vi "Autonomous Independent.vi"() -> ()   [LabVIEW 2012]
doc: "This VI is called when autonomous begins, and will automatically be terminated when autonomous ends. You can carry out timed or sensor driven robot movement independently without needing to return to the caller."
uses:
  Auto States.ctl
  <vilib>/Rock Robotics/WPI/Relay/WPI_RelayValue.ctl
  <vilib>/Rock Robotics/WPI/Solenoid/WPI_SolenoidValue.ctl
  Robot Global Data.vi
  <vilib>/Rock Robotics/WPI/RobotDrive/WPI_RobotDriveGetSetRefNum.vi
  <vilib>/Rock Robotics/WPI/Solenoid/WPI_SolenoidSetEnum.vi
  <vilib>/Rock Robotics/WPI/RobotDrive/WPI_RobotDriveArcadeDrive_Standard(NoSaturation).vi
panel:
  in  "Debug":bool
  in  "?":T1
  out "Current Movement, for debugging":T2 {"Y Joystick Value" scale=1.0..-1.0; "X Joystick Value" scale=-1.0..1.0}
  in  "Array of robot movements":T3(array[cluster]) {"Y Joystick Value" scale=1.0..-1.0; "X Joystick Value" scale=-1.0..1.0}
  # "Be sure to right-click and choose Data Operations>>Make Current Value default if you want to save the array values with the VI"
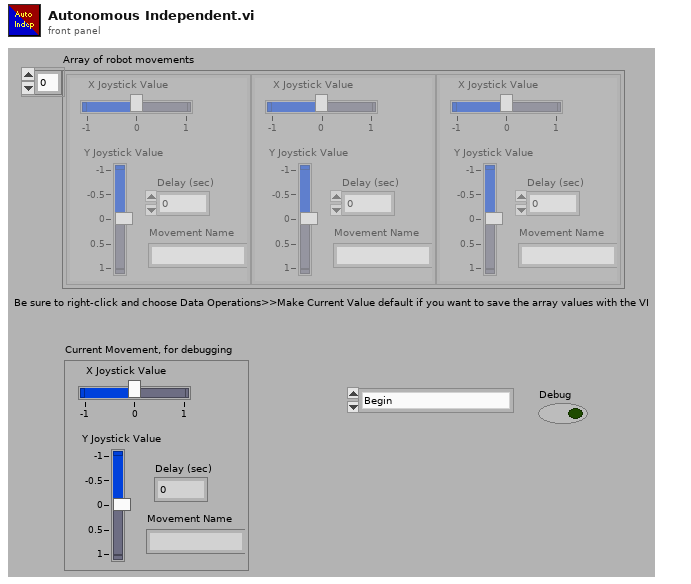
[diagram p1: front panel]
types:
  T1 = typedef "Auto States.ctl" = enum16{"Begin", "2 Top/Mid Goal", "3 Top/Mid Goal", "Drive to shoot", "Auto-Lock", "Spin 180 and Auto-Lock", "Drive Backwards", "Drive forward (Dump)", "Slow Shoot", "End"}
  T2 = cluster{"X Joystick Value":dbl, "Y Joystick Value":dbl, "Delay (sec)":dbl, "Movement Name":string}
  T3 = cluster{"X Joystick Value":dbl, "Y Joystick Value":dbl, "Delay (sec)":dbl, "Movement Name":string}[]
  T4 = typedef "WPI_RobotDriveDevRef.ctl" = cluster{"DevStatus":errorcluster, "Motors[]":T5[], "Square Inputs":bool, "Max Output":dbl, "Isochronous":bool}
  T5 = typedef "WPI_MotorControlDeviceRef.ctl" = cluster{"DeviceStatus":errorcluster, "Type":enum16{"PWM", "CAN"}, "PWM":cluster{"Digital Module":T6, "PWM Channel":T7, "DeadBand":T8}, "CAN":cluster{"Device Number":u8, "Control Mode":T9, "Semaphore":T10, "Max Vout":dbl}, "Invert":bool, "TransformRef":T11, "InvTransformRef":T11}
  T6 = typedef "FPGA_TypedefDigitalModule.ctl" = enum16{"Digital Module 1", "Digital Module 2"}
  T7 = typedef "FPGA_DIOPWMChannel.ctl" = enum8{"PWM 1", "PWM 2", "PWM 3", "PWM 4", "PWM 5", "PWM 6", "PWM 7", "PWM 8", "PWM 9", "PWM 10", "Invalid"}
  T8 = typedef "WPI_PWMDeadband.ctl" = cluster{"Name":string, "maxPositivePwm":i32, "minPositivePwm":i32, "centerPwm":i32, "maxNegativePwm":i32, "minNegativePwm":i32, "angularRange":u16}
  T9 = typedef "WPI_CANJaguar_ControlMode.ctl" = enum8{"Percent VBus", "Current", "Speed", "Position", "Voltage"}
  T10 = typedef "Semaphore RefNum" = refnum<k1>
  T11 = typedef "WPI_PWMTransform_ConPane.ctl" = refnum<vi>
  T12 = typedef "Auto State Selector.ctl" = enum16{"None", "Fire 2x", "Fire 3x", "Fire 3x from back", "Dump in low goal"}
  T13 = typedef "WPI_RelayValue.ctl" = enum16{"Off", "On", "Forward", "Reverse"}
  T14 = typedef "WPI_SolenoidValue.ctl" = enum16{"Off", "On", "Forward", "Reverse"}
  T15 = typedef "WPI_RelayDevRef.ctl" = cluster{"DevStatus":errorcluster, "Relay Channel":T16, "Digital Module":T6, "Relay Direction":T17}
  T16 = typedef "FPGA_DIORelayChannel.ctl" = enum8{"Relay 1", "Relay 2", "Relay 3", "Relay 4", "Relay 5", "Relay 6", "Relay 7", "Relay 8", "Invalid"}
  T17 = typedef "WPI_RelayDirection.ctl" = enum16{"Both directions", "Forward only", "Reverse only"}
  T18 = typedef "WPI_SolenoidDevRef.ctl" = cluster{"DevStatus":errorcluster, "Solenoid Module":T19, "Forward Solenoid Channel":T20, "Reverse Solenoid Channel":T20}
  T19 = typedef "FPGA_TypedefSolenoidModule.ctl" = enum16{"Solenoid Module 1", "Solenoid Module 2"}
  T20 = typedef "WPI_SolenoidChannel.ctl" = enum8{"Solenoid 1", "Solenoid 2", "Solenoid 3", "Solenoid 4", "Solenoid 5", "Solenoid 6", "Solenoid 7", "Solenoid 8", "Invalid"}
  T21 = cluster{"Center Position":cluster{"X":dbl, "Y":dbl}, "Distance (ft)":dbl, "Center":bool, "Top":bool, "Mid":bool}[]
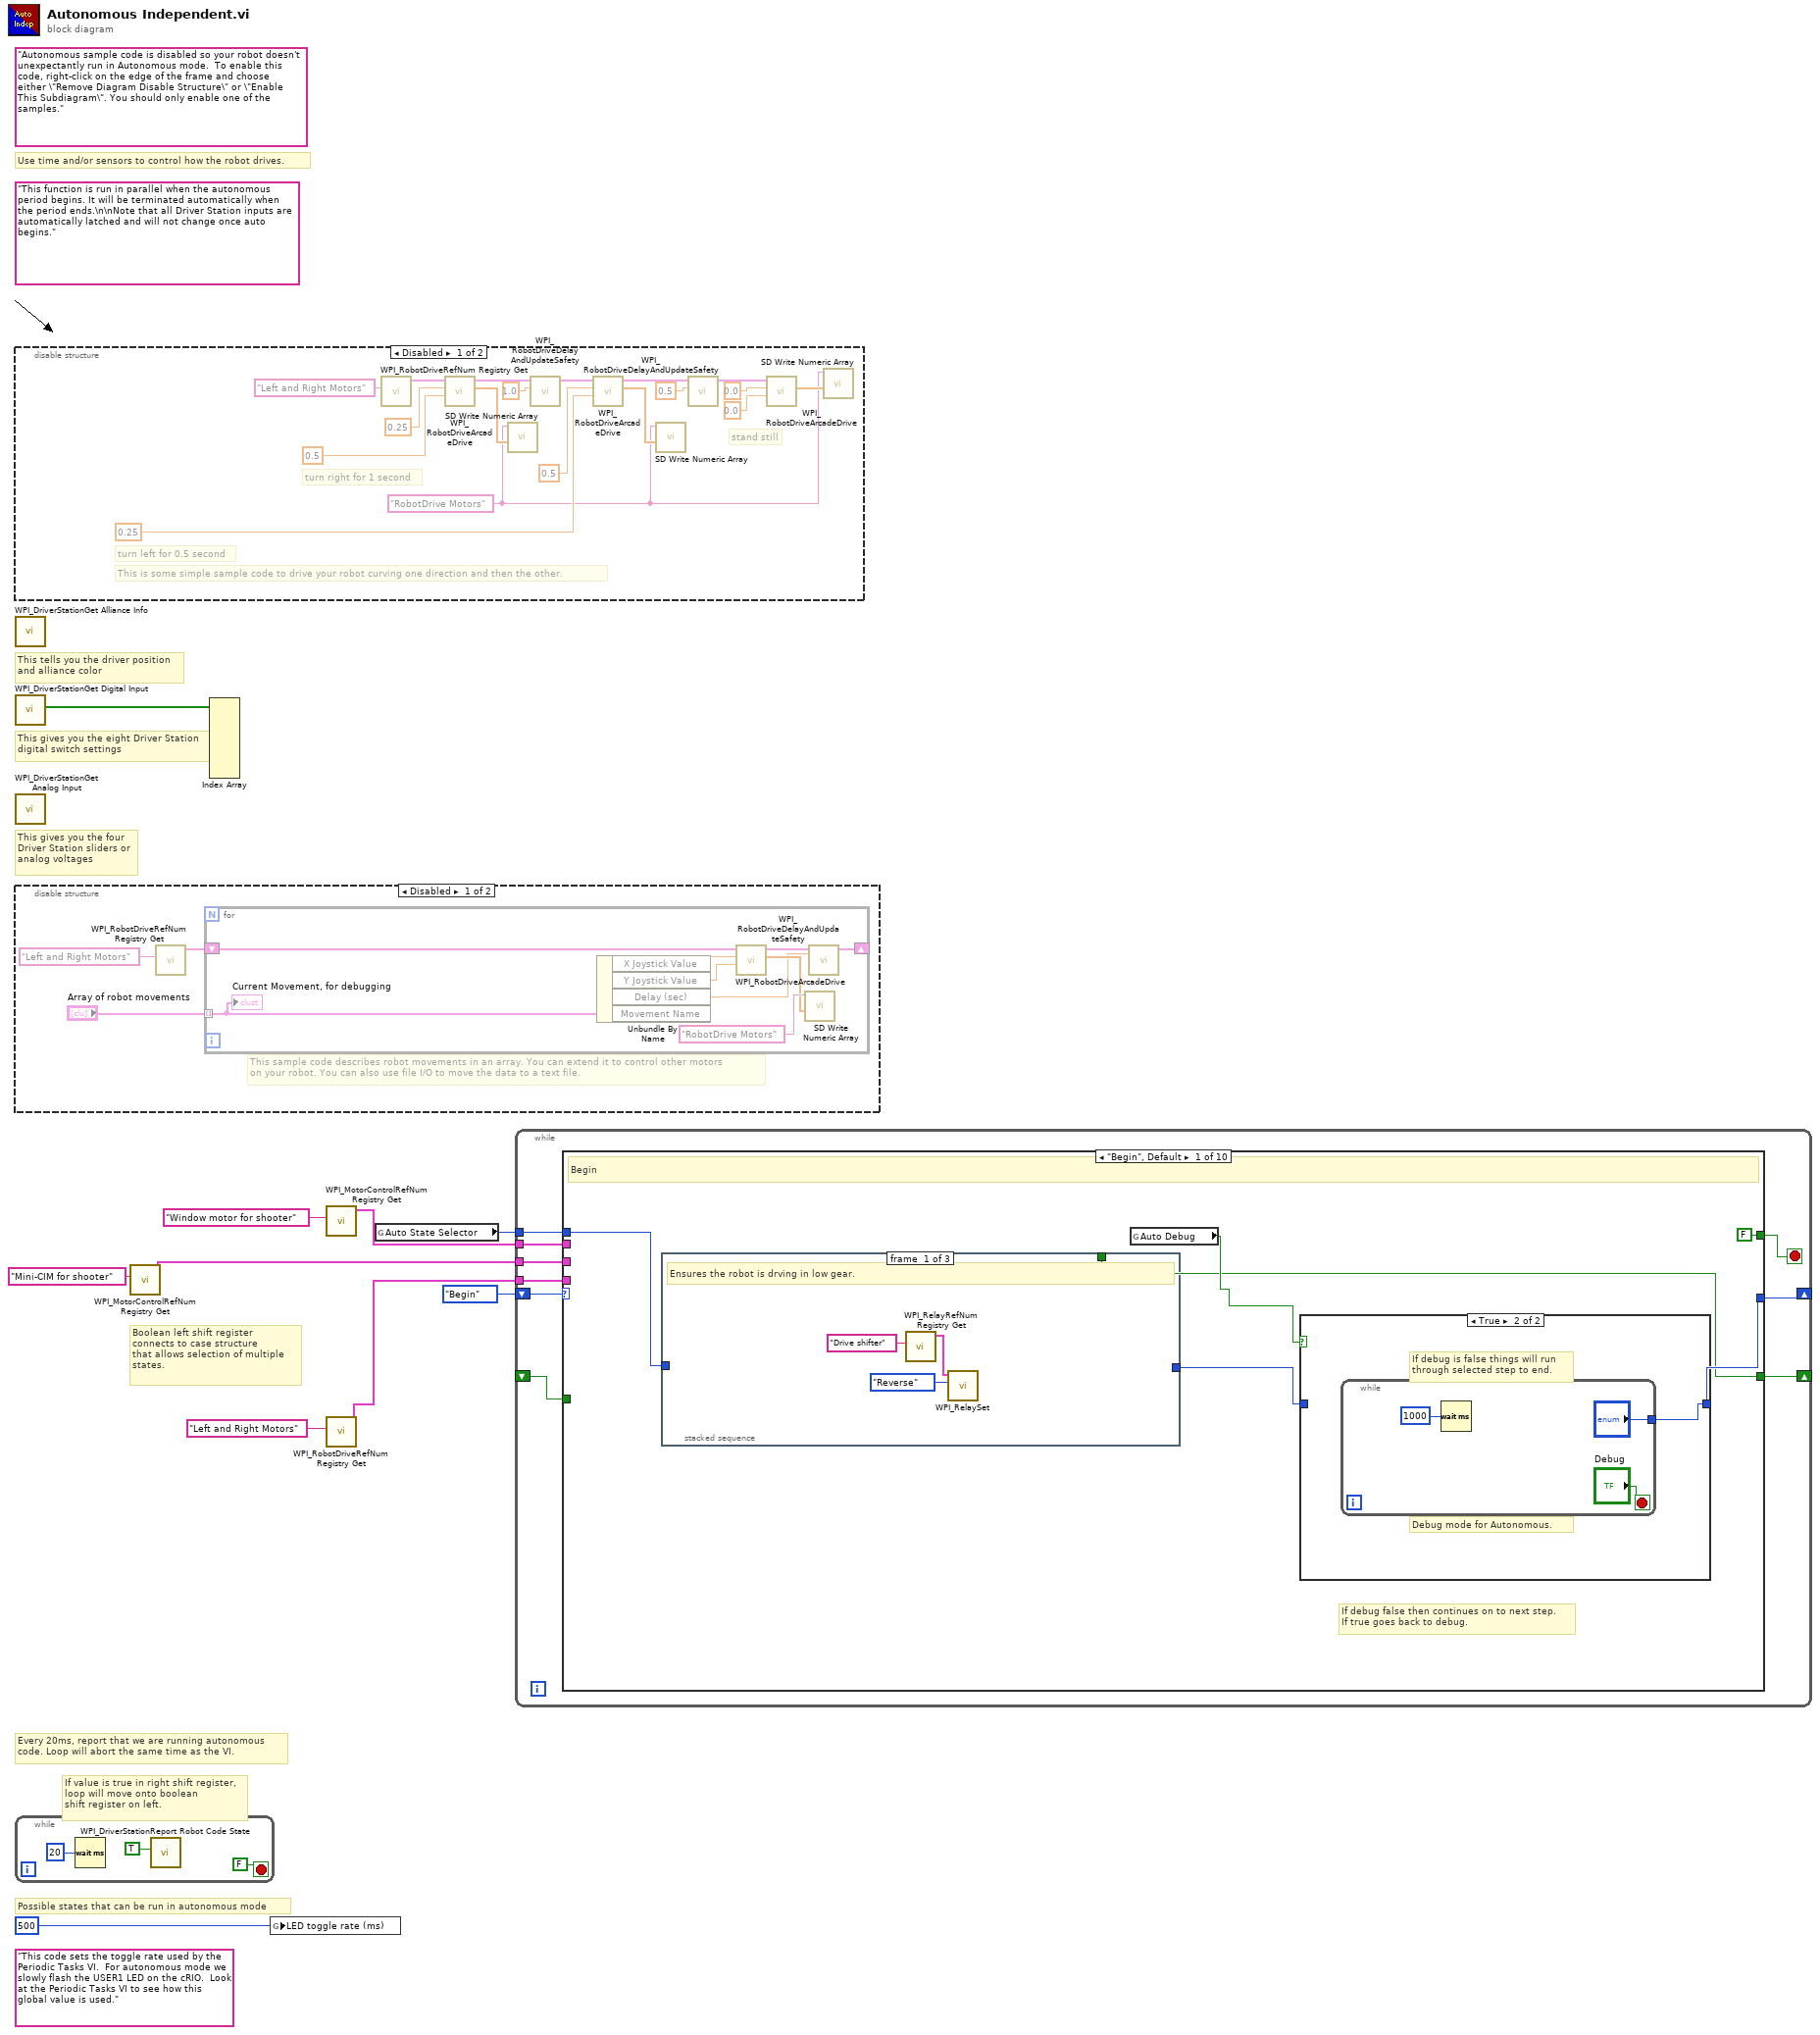
[diagram p0: block diagram]
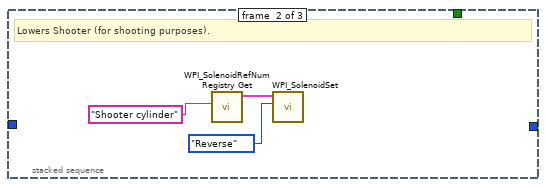
[diagram p2: hidden frame]
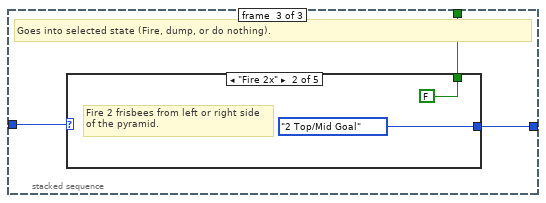
[diagram p3: hidden frame]
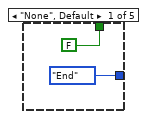
[diagram p4: hidden frame]
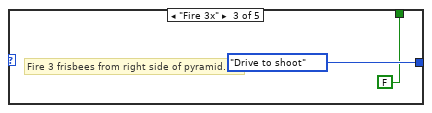
[diagram p5: hidden frame]
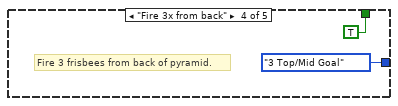
[diagram p6: hidden frame]
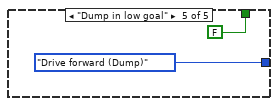
[diagram p7: hidden frame]
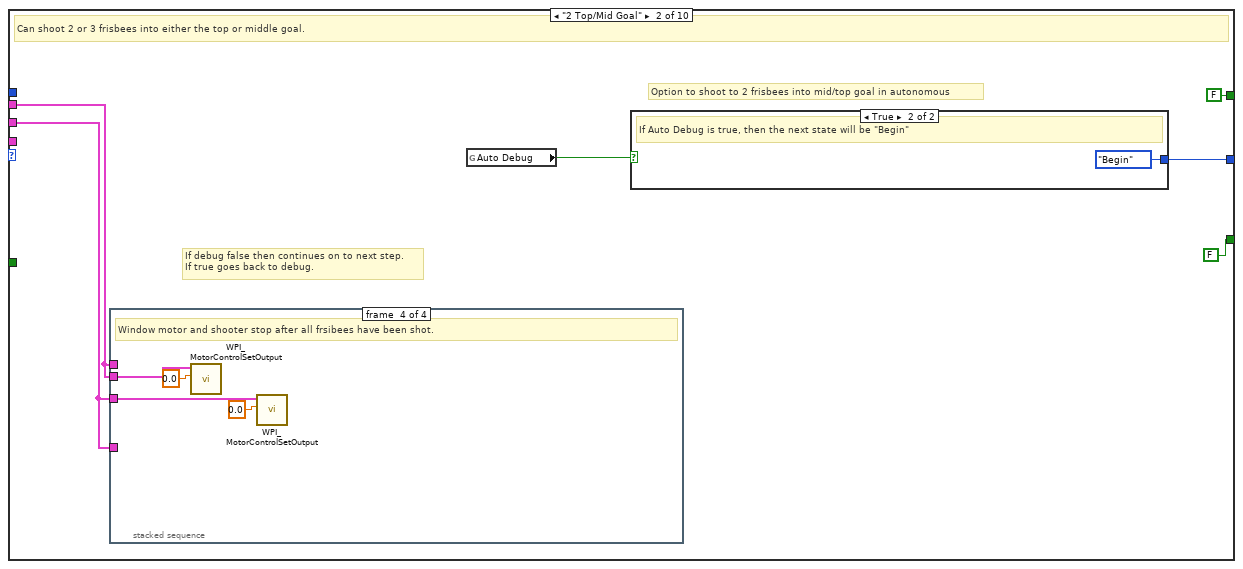
[diagram p9: hidden frame]
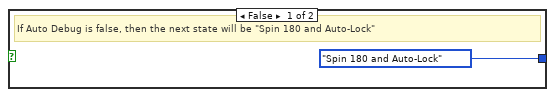
[diagram p10: hidden frame]
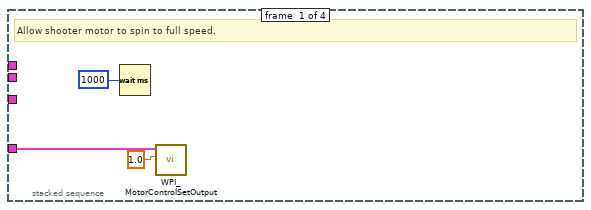
[diagram p11: hidden frame]
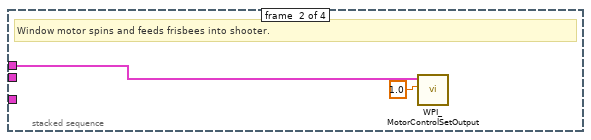
[diagram p12: hidden frame]
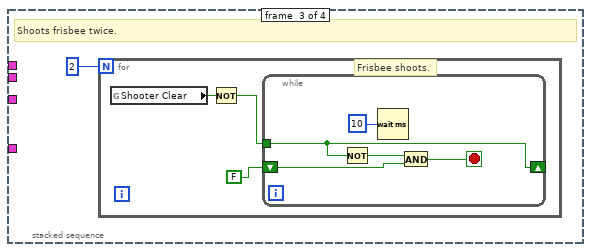
[diagram p13: hidden frame]
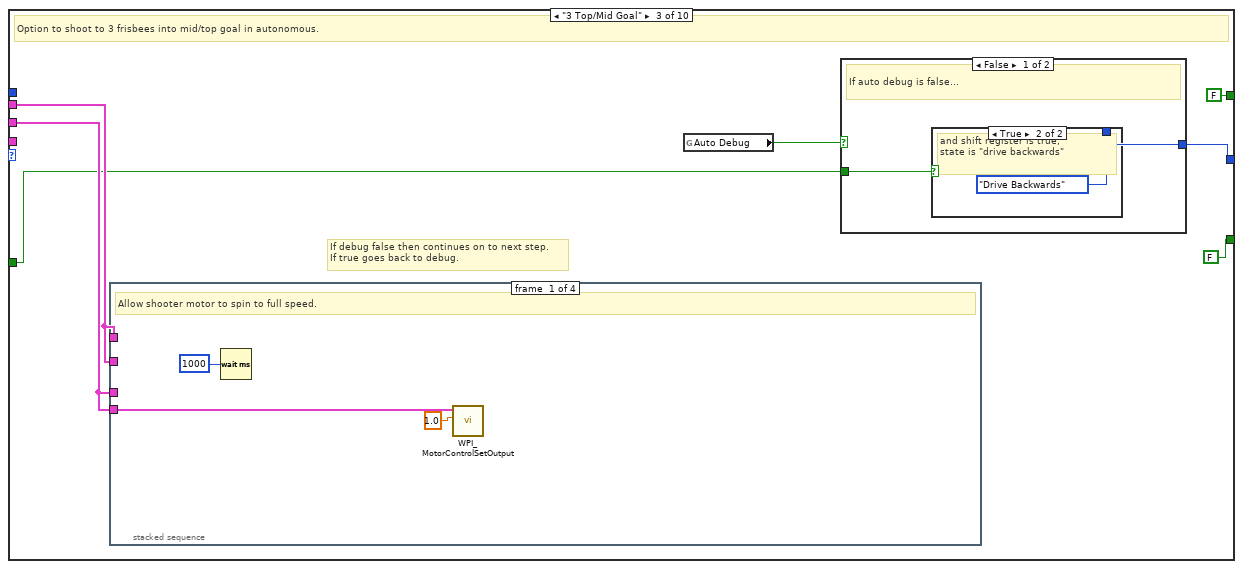
[diagram p14: hidden frame]
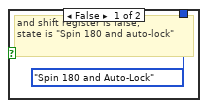
[diagram p15: hidden frame]
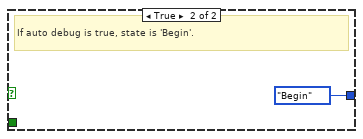
[diagram p16: hidden frame]
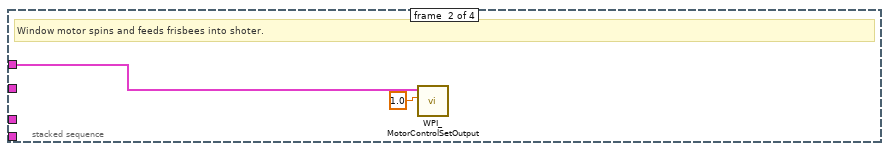
[diagram p17: hidden frame]
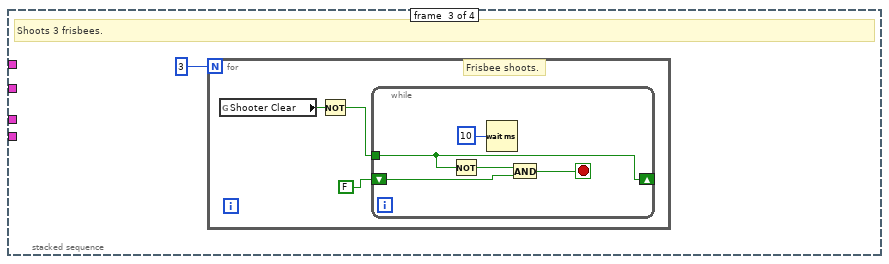
[diagram p18: hidden frame]
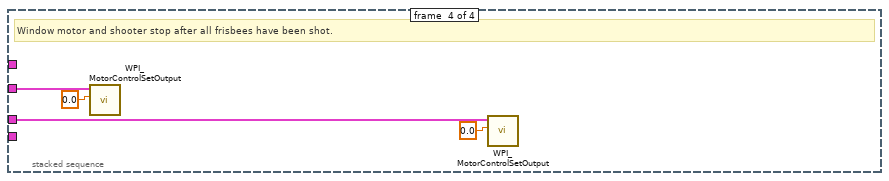
[diagram p19: hidden frame]
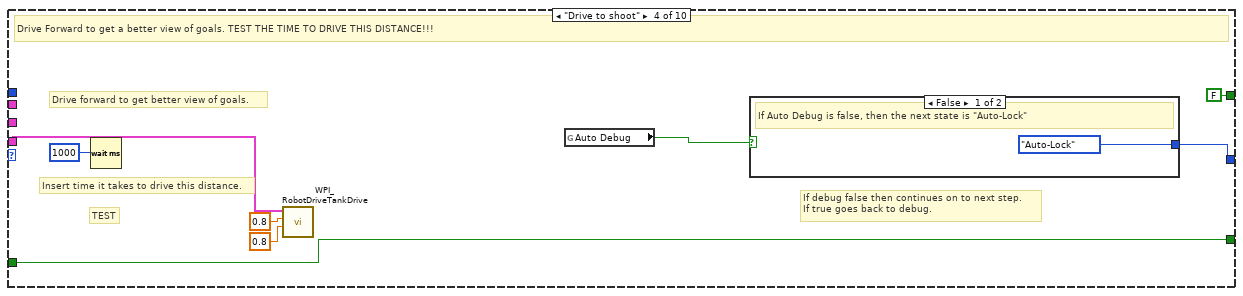
[diagram p20: hidden frame]
diagram:
  (unwired) "This code sets the toggle rate used by the Periodic Tasks VI.  For autonomous mode we slowly flash the USER1 LED on the cRIO.  Look at the Periodic Tasks VI to see how this global value is used."
  (unwired) "Autonomous sample code is disabled so your robot doesn't unexpectantly run in Autonomous mode.  To enable this code, right-click on the edge of the frame and choose either \"Remove Diagram Disable Structure\" or \"Enable This Subdiagram\". You should only enable one of the samples."
  (unwired) "This function is run in parallel when the autonomous period begins. It will be terminated automatically when the period ends.\n\nNote that all Driver Station inputs are automatically latched and will not change once auto begins."
  # "Boolean left shift register\nconnects to case structure\nthat allows selection of multiple \nstates."
  # "If value is true in right shift register,\nloop will move onto boolean\nshift register on left."
  # "Possible states that can be run in autonomous mode"
  # "Every 20ms, report that we are running autonomous\ncode. Loop will abort the same time as the VI."
  # "Use time and/or sensors to control how the robot drives."
  # "This tells you the driver position\nand alliance color"
  # "This gives you the eight Driver Station\ndigital switch settings"
  # "This gives you the four\nDriver Station sliders or\nanalog voltages"
  n1 = disable-structure shown="Disabled" {
    frame Disabled {
      w11 = "RobotDrive Motors" ("Name")
      # "This is some simple sample code to drive your robot curving one direction and then the other."
      # "stand still"
      # "turn left for 0.5 second"
      # "turn right for 1 second"
      n2 = call <vilib>:"WPI_RobotDriveRefNum Registry Get.vi"("refnum name"="Left and Right Motors") -> ("RobotDriveDevRef"=w15:T4)  [unwired: 1 in, 9 out]
      n3 = call-poly <vilib>:"WPI_RobotDriveArcadeDrive.vi"("Y axis value"=0.5 ("X axis value"), "X axis value"=0.25, "RobotDriveDevRef"=w15) -> ("Motor Values"=w14:dbl[], "RobotDriveDevRef"=w22:T4)  [unwired: 1 in, 6 out]
      n4 = call <vilib>:"SD Write Numeric Array.vi"("Numeric Array"=w14, "Name"=w11) -> ()  [unwired: 8 in, 2 out]
      n5 = call <vilib>:"WPI_RobotDriveDelayAndUpdateSafety.vi"("Delay (s)"=1.0, "RobotDriveDevRef"=w22) -> ("RobotDriveDevRef 2"=w21:T4)  [unwired: 8 in, 1 out]
      n6 = call-poly <vilib>:"WPI_RobotDriveArcadeDrive.vi"("Y axis value"=0.25 ("X axis value"), "X axis value"=0.5, "RobotDriveDevRef"=w21) -> ("Motor Values"=w13:dbl[], "RobotDriveDevRef"=w20:T4)  [unwired: 1 in, 6 out]
      n7 = call <vilib>:"SD Write Numeric Array.vi"("Numeric Array"=w13, "Name"=w11) -> ()  [unwired: 8 in, 2 out]
      n8 = call <vilib>:"WPI_RobotDriveDelayAndUpdateSafety.vi"("Delay (s)"=0.5, "RobotDriveDevRef"=w20) -> ("RobotDriveDevRef 2"=w19:T4)  [unwired: 8 in, 1 out]
      n9 = call-poly <vilib>:"WPI_RobotDriveArcadeDrive.vi"("Y axis value"=0.0 ("X axis value"), "X axis value"=0.0, "RobotDriveDevRef"=w19) -> ("Motor Values"=w12:dbl[])  [unwired: 1 in, 7 out]
      n10 = call <vilib>:"SD Write Numeric Array.vi"("Numeric Array"=w12, "Name"=w11) -> ()  [unwired: 8 in, 2 out]
    }
    frame Enabled {
    }
  }
  n11 = call <vilib>:"WPI_DriverStationGet Alliance Info.vi"() -> ()  [unwired: 12 out]
  n12 = call <vilib>:"WPI_DriverStationGet Digital Input.vi"() -> ("Driver Station Digital Input (1-8)"=w10:bool[])  [unwired: 11 out]
  n13 = call <vilib>:"WPI_DriverStationGet Analog Input.vi"() -> ()  [unwired: 12 out]
  n14 = disable-structure shown="Disabled" {
    frame Disabled {
      # "This sample code describes robot movements in an array. You can extend it to control other motors\non your robot. You can also use file I/O to move the data to a text file."
      n15 = call <vilib>:"WPI_RobotDriveRefNum Registry Get.vi"("refnum name"="Left and Right Motors") -> ("RobotDriveDevRef"=w30:T4)  [unwired: 1 in, 9 out]
      n16 = for {
        shift-right: [w36] -> _
        shift-left: w30 -> [w37]
        tunnel: "Array of robot movements" -> [w32] mode=indexing
        n17 = Unbundle By Name(w32) -> ("X Joystick Value"=w35:dbl, "Y Joystick Value"=w34:dbl, "Delay (sec)"=w33:dbl)  [unwired: 1 out]
        n18 = call-poly <vilib>:"WPI_RobotDriveArcadeDrive.vi"("Y axis value"=w34, "X axis value"=w35, "RobotDriveDevRef"=w37) -> ("Motor Values"=w39:dbl[], "RobotDriveDevRef"=w38:T4)  [unwired: 1 in, 6 out]
        n19 = call <vilib>:"SD Write Numeric Array.vi"("Numeric Array"=w39, "Name"="RobotDrive Motors") -> ()  [unwired: 8 in, 2 out]
        n20 = call <vilib>:"WPI_RobotDriveDelayAndUpdateSafety.vi"("Delay (s)"=w33, "RobotDriveDevRef"=w38) -> ("RobotDriveDevRef 2"=w36:T4)  [unwired: 8 in, 1 out]
        "Current Movement, for debugging" <- w32
      }
    }
    frame Enabled {
    }
  }
  n21 = while {
    stop <- FALSE stop-if-true
    n22 = Wait (ms)(milliseconds to wait=u32 20) -> ()  [unwired: 1 out]
    n23 = call <vilib>:"WPI_DriverStationReport Robot Code State.vi"("Autonomous"=TRUE) -> ()  [unwired: 10 in, 1 out]
  }
  n24 = call <vilib>:"WPI_MotorControlRefNum Registry Get.vi"("refnum name"="Mini-CIM for shooter") -> ("MotorControlDevRef"=w5:T5)  [unwired: 9 in, 1 out]
  n25 = Index Array(array=w10) -> ()  [unwired: 8 in, 8 out]
  n26 = global write "Robot Global Data.vi" "LED toggle rate (ms)"(u32 500 ("LED ms toggle rate")) -> ()
  n27 = call <vilib>:"WPI_MotorControlRefNum Registry Get.vi"("refnum name"="Window motor for shooter") -> ("MotorControlDevRef"=w4:T5)  [unwired: 9 in, 1 out]
  n28 = call <vilib>:"WPI_RobotDriveRefNum Registry Get.vi"("refnum name"="Left and Right Motors") -> ("RobotDriveDevRef"=w2:T4)  [unwired: 1 in, 9 out]
  n29 = global read "Robot Global Data.vi" "Auto State Selector"() -> (w1:T12)
  n30 = while {
    shift-right: [w52] -> _
    shift-left: Auto_States."Begin" -> [w46]
    tunnel: w5 -> [w51]
    tunnel: w4 -> [w48]
    tunnel: w2 -> [w49]
    tunnel: w1 -> [w47]
    shift-right: [w45] -> _
    shift-left: _ -> [w44]
    stop <- w50 stop-if-true
    n31 = case shown="\"Begin\", Default" w46 {
      tunnel: [w57 w85 w112 w144 w154 w162 w182 w193 w202 w226] -> w52
      tunnel: w51 -> [_ w86 w113 _ _ _ _ _ w199 _]
      tunnel: [FALSE FALSE FALSE FALSE FALSE FALSE FALSE FALSE FALSE TRUE] -> w50
      tunnel: w49 -> [_ _ _ w145 _ w164 w179 w191 _ _]
      tunnel: w48 -> [_ w87 w114 _ _ _ _ _ w200 _]
      tunnel: w47 -> [w55 _ _ _ _ _ _ _ _ _]
      tunnel: [w53 FALSE FALSE w139 FALSE FALSE FALSE FALSE FALSE FALSE] -> w45
      tunnel: w44 -> [_ _ w109 w139 w150 _ _ _ _ _]
      frame "Begin", Default {
        # "If debug false then continues on to next step.\nIf true goes back to debug."
        # "Begin"
        n32 = stacked-sequence {
          tunnel: w55 -> [_ _ w67]
          tunnel: [_ _ w66] -> w54
          tunnel: [_ _ w65] -> w53
          frame #0 {
            # "Ensures the robot is drving in low gear."
            n33 = call <vilib>:"WPI_RelayRefNum Registry Get.vi"("refnum name"="Drive shifter") -> ("RelayDevRef"=w59:T15)  [unwired: 9 in, 1 out]
            n34 = call <vilib>:"WPI_RelaySet.vi"("RelayValue"=WPI_RelayValue."Reverse", "RelayDevRef"=w59) -> ()  [unwired: 8 in, 2 out]
          }
          frame #1 {
            # "Lowers Shooter (for shooting purposes)."
            n35 = call <vilib>:"WPI_SolenoidRefNum Registry Get.vi"("refnum name"="Shooter cylinder") -> ("SolenoidDevRef"=w63:T18)  [unwired: 9 in, 1 out]
            n36 = call-poly <vilib>:"WPI_SolenoidSet.vi"("Value"=WPI_SolenoidValue."Reverse", "SolenoidDevRef"=w63) -> ()  [unwired: 8 in, 2 out]
          }
          frame #2 {
            # "Goes into selected state (Fire, dump, or do nothing)."
            n37 = case shown="\"Fire 2x\"" w67 {
              tunnel: [Auto_States."End" Auto_States."2 Top/Mid Goal" Auto_States."Drive to shoot" Auto_States."3 Top/Mid Goal" Auto_States."Drive forward (Dump)"] -> w66
              tunnel: [FALSE FALSE FALSE TRUE FALSE] -> w65
              frame "None", Default {
              }
              frame "Fire 2x" {
                # "Fire 2 frisbees from left or right side\nof the pyramid."
              }
              frame "Fire 3x" {
                # "Fire 3 frisbees from right side of pyramid."
              }
              frame "Fire 3x from back" {
                # "Fire 3 frisbees from back of pyramid."
              }
              frame "Dump in low goal" {
              }
            }
          }
        }
        n38 = global read "Robot Global Data.vi" "Auto Debug"() -> (w56:bool)
        n39 = case shown="True" w56 {
          tunnel: [w78 w79] -> w57
          tunnel: w54 -> [w78 _]
          frame False {
          }
          frame True {
            # "If debug is false things will run \nthrough selected step to end."
            # "Debug mode for Autonomous."
            n40 = while {
              tunnel: ["?"] -> w79
              stop <- "Debug" stop-if-true
              n41 = Wait (ms)(milliseconds to wait=u32 1000) -> ()  [unwired: 1 out]
            }
          }
        }
      }
      frame "2 Top/Mid Goal" {
        # "If debug false then continues on to next step.\nIf true goes back to debug."
        # "Option to shoot to 2 frisbees into mid/top goal in autonomous"
        # "Can shoot 2 or 3 frisbees into either the top or middle goal."
        n42 = stacked-sequence {
          tunnel: w86 -> [w93 _ _ _]
          tunnel: w87 -> [_ w94 _ _]
          tunnel: w87 -> [_ _ _ w106]
          tunnel: w86 -> [_ _ _ w105]
          frame #0 {
            # "Allow shooter motor to spin to full speed."
            n43 = Wait (ms)(milliseconds to wait=u32 1000) -> ()  [unwired: 1 out]
            n44 = call <vilib>:"WPI_MotorControlSetOutput.vi"("Output"=1.0, "MotorControlDevRef"=w93) -> ()  [unwired: 7 in, 3 out]
          }
          frame #1 {
            # "Window motor spins and feeds frisbees into shooter."
            n45 = call <vilib>:"WPI_MotorControlSetOutput.vi"("Output"=1.0, "MotorControlDevRef"=w94) -> ()  [unwired: 7 in, 3 out]
          }
          frame #2 {
            # "Shoots frisbee twice."
            n46 = for {
              N: 2 -> [_]
              # "Frisbee shoots."
              n47 = global read "Robot Global Data.vi" "Shooter Clear"() -> (w99:bool)
              n48 = Not(x=w99) -> (.not. x?=w98:bool)
              n49 = while {
                shift-right: [w101] -> _
                shift-left: FALSE -> [w103]
                tunnel: w98 -> [w101]
                stop <- w100 stop-if-true
                n50 = Not(x=w101) -> (.not. x?=w102:bool)
                n51 = Wait (ms)(milliseconds to wait=u32 10 ("millisecond timer value")) -> ()  [unwired: 1 out]
                n52 = And(x=w102, y=w103) -> (x .and. y?=w100:bool)
              }
            }
          }
          frame #3 {
            # "Window motor and shooter stop after all frsibees have been shot."
            n53 = call <vilib>:"WPI_MotorControlSetOutput.vi"("Output"=0.0, "MotorControlDevRef"=w106) -> ()  [unwired: 7 in, 3 out]
            n54 = call <vilib>:"WPI_MotorControlSetOutput.vi"("Output"=0.0, "MotorControlDevRef"=w105) -> ()  [unwired: 7 in, 3 out]
          }
        }
        n55 = global read "Robot Global Data.vi" "Auto Debug"() -> (w84:bool)
        n56 = case shown="True" w84 {
          tunnel: [Auto_States."Spin 180 and Auto-Lock" Auto_States."Begin"] -> w85
          frame False {
            # "If Auto Debug is false, then the next state will be \"Spin 180 and Auto-Lock\""
          }
          frame True {
            # "If Auto Debug is true, then the next state will be \"Begin\""
          }
        }
      }
      frame "3 Top/Mid Goal" {
        # "If debug false then continues on to next step.\nIf true goes back to debug."
        # "Option to shoot to 3 frisbees into mid/top goal in autonomous."
        n57 = stacked-sequence {
          tunnel: w113 -> [w123 _ _ _]
          tunnel: w114 -> [_ w124 _ _]
          tunnel: w114 -> [_ _ _ w136]
          tunnel: w113 -> [_ _ _ w135]
          frame #0 {
            # "Allow shooter motor to spin to full speed."
            n58 = Wait (ms)(milliseconds to wait=u32 1000) -> ()  [unwired: 1 out]
            n59 = call <vilib>:"WPI_MotorControlSetOutput.vi"("Output"=1.0, "MotorControlDevRef"=w123) -> ()  [unwired: 7 in, 3 out]
          }
          frame #1 {
            # "Window motor spins and feeds frisbees into shoter."
            n60 = call <vilib>:"WPI_MotorControlSetOutput.vi"("Output"=1.0, "MotorControlDevRef"=w124) -> ()  [unwired: 7 in, 3 out]
          }
          frame #2 {
            # "Shoots 3 frisbees."
            n61 = for {
              N: 3 -> [_]
              # "Frisbee shoots."
              n62 = global read "Robot Global Data.vi" "Shooter Clear"() -> (w129:bool)
              n63 = Not(x=w129) -> (.not. x?=w128:bool)
              n64 = while {
                shift-right: [w131] -> _
                shift-left: FALSE -> [w133]
                tunnel: w128 -> [w131]
                stop <- w130 stop-if-true
                n65 = Not(x=w131) -> (.not. x?=w132:bool)
                n66 = Wait (ms)(milliseconds to wait=u32 10 ("millisecond timer value")) -> ()  [unwired: 1 out]
                n67 = And(x=w132, y=w133) -> (x .and. y?=w130:bool)
              }
            }
          }
          frame #3 {
            # "Window motor and shooter stop after all frisbees have been shot."
            n68 = call <vilib>:"WPI_MotorControlSetOutput.vi"("Output"=0.0, "MotorControlDevRef"=w136) -> ()  [unwired: 7 in, 3 out]
            n69 = call <vilib>:"WPI_MotorControlSetOutput.vi"("Output"=0.0, "MotorControlDevRef"=w135) -> ()  [unwired: 7 in, 3 out]
          }
        }
        n70 = global read "Robot Global Data.vi" "Auto Debug"() -> (w111:bool)
        n71 = case shown="False" w111 {
          tunnel: [w117 Auto_States."Begin"] -> w112
          tunnel: w109 -> [w116 _]
          frame False {
            # "If auto debug is false..."
            n72 = case shown="True" w116 {
              tunnel: [Auto_States."Spin 180 and Auto-Lock" Auto_States."Drive Backwards"] -> w117
              frame False {
                # "and shift register is false, \nstate is \"Spin 180 and auto-lock\""
              }
              frame True {
                # "and shift register is true,\nstate is \"drive backwards\""
              }
            }
          }
          frame True {
            # "If auto debug is true, state is 'Begin'."
          }
        }
      }
      frame "Drive to shoot" {
        # "TEST"
        # "Insert time it takes to drive this distance."
        # "If debug false then continues on to next step.\nIf true goes back to debug."
        # "Drive forward to get better view of goals."
        # "Drive Forward to get a better view of goals. TEST THE TIME TO DRIVE THIS DISTANCE!!!"
        n73 = Wait (ms)(milliseconds to wait=u32 1000) -> ()  [unwired: 1 out]
        n74 = call <vilib>:"WPI_RobotDriveTankDrive.vi"("Right axis value"=0.8, "Left axis value"=0.8, "RobotDriveDevRef"=w145) -> ()  [unwired: 6 in, 3 out]
        n75 = global read "Robot Global Data.vi" "Auto Debug"() -> (w140:bool)
        n76 = case shown="False" w140 {
          tunnel: [Auto_States."Auto-Lock" Auto_States."Begin"] -> w144
          frame False {
            # "If Auto Debug is false, then the next state is \"Auto-Lock\""
          }
          frame True {
            # "If Auto Debug is true, then the next state is \"Begin\""
          }
        }
      }
      frame "Auto-Lock" {
        # "If debug false then continues on to next step.\nIf true goes back to debug."
        # "When robot pivots it will stop when it auto-locks on goal."
        n77 = global write "Robot Global Data.vi" "Auto-lock"(TRUE) -> ()
        n78 = global read "Robot Global Data.vi" "Auto Debug"() -> (w152:bool)
        n79 = case shown="False" w152 {
          tunnel: [w156 Auto_States."Begin"] -> w154
          tunnel: w150 -> [w155 _]
          frame False {
            # "If Auto Debug is false..."
            n80 = case shown="False" w155 {
              tunnel: [Auto_States."2 Top/Mid Goal" Auto_States."3 Top/Mid Goal"] -> w156
              frame False {
                # "Fires 2 discs into goal."
              }
              frame True {
                # "Fires 3 frisbees in goal"
              }
            }
          }
          frame True {
            # "If Auto Debug is true, then the next state is \"Begin\""
          }
        }
      }
      frame "Spin 180 and Auto-Lock" {
        # "If debug false then continues on to next step.\nIf true goes back to debug."
        # "Robot spins 180 degrees (losing auto-lock from ally goal) and locks onto opponent goal."
        n81 = stacked-sequence {
          tunnel: w164 -> [w168 _ _]
          tunnel: w164 -> [_ _ _]
          frame #0 {
            # "Robot will spin 180 degrees (Dead Reckon)"
            n82 = call <vilib>:"WPI_RobotDriveTankDrive.vi"("Right axis value"=-1.0, "Left axis value"=1.0, "RobotDriveDevRef"=w168) -> ()  [unwired: 6 in, 3 out]
            n83 = Wait (ms)(milliseconds to wait=u32 3000) -> ()  [unwired: 1 out]
          }
          frame #1 {
            # "When Robot pivots it will stop when it auto-locks onto goal."
            n84 = global write "Robot Global Data.vi" "Auto-lock"(TRUE) -> ()
          }
          frame #2 {
            # "continue when any target is found"
            n85 = while {
              stop <- w173 stop-if-true
              n86 = global read "Robot Global Data.vi" "Target Info"() -> (w176:T21)
              n87 = Array Size(array=w176) -> (size(s)=w175:i32)
              n88 = Wait (ms)(milliseconds to wait=u32 1000) -> ()  [unwired: 1 out]
              n89 = Greater?(x=w175, y=0) -> (0:w173:bool)
            }
          }
        }
        n90 = global read "Robot Global Data.vi" "Auto Debug"() -> (w161:bool)
        n91 = case shown="False" w161 {
          tunnel: [Auto_States."End" Auto_States."Begin"] -> w162
          frame False {
            # "If Auto Debug is false, then the next state is \"End\""
          }
          frame True {
            # "If Auto Debug is true, then the next state is \"Begin\""
          }
        }
      }
      frame "Drive Backwards" {
        # "Amount of time it takes to back up a little."
        # "Make robot drive backwards so it may be able to turn 180 degrees."
        n92 = call <vilib>:"WPI_RobotDriveTankDrive.vi"("Right axis value"=-0.3, "Left axis value"=-0.3, "RobotDriveDevRef"=w179) -> ()  [unwired: 6 in, 3 out]
        n93 = Wait (ms)(milliseconds to wait=u32 2000) -> ()  [unwired: 1 out]
        n94 = global read "Robot Global Data.vi" "Auto Debug"() -> (w177:bool)
        n95 = case shown="True" w177 {
          tunnel: [Auto_States."Spin 180 and Auto-Lock" Auto_States."Begin"] -> w182
          frame False {
            # "If Auto Debug is false, then the next state is \"Spin 180 and Auto-Lock\""
          }
          frame True {
            # "If Auto Debug is true, then the next state is \"Begin\""
          }
        }
      }
      frame "Drive forward (Dump)" {
        # "Time is the estimated time it takes to get to \nlow goal."
        # "Robot drives backward slowly until it is up against the low goal."
        n96 = call <vilib>:"WPI_RobotDriveTankDrive.vi"("Right axis value"=0.3, "Left axis value"=0.3, "RobotDriveDevRef"=w191) -> ()  [unwired: 6 in, 3 out]
        n97 = Wait (ms)(milliseconds to wait=u32 5000) -> ()  [unwired: 1 out]
        n98 = global read "Robot Global Data.vi" "Auto Debug"() -> (w192:bool)
        n99 = case shown="False" w192 {
          tunnel: [Auto_States."Slow Shoot" Auto_States."Begin"] -> w193
          frame False {
            # "If Auto Debug is false, then the next state is \"Slow Shoot\""
          }
          frame True {
            # "If Auto Debug is true, then the next state is \"Begin\""
          }
        }
      }
      frame "Slow Shoot" {
        # "When Dumping, use \"Slow Shoot\" to fire slowly into the lowest goal."
        n100 = stacked-sequence {
          tunnel: w200 -> [_ w208 _ w220]
          tunnel: w199 -> [w205 _ _ w219]
          frame #0 {
            # "Allow shooter motor\n to spin to slow speed."
            # "Sensor will determine how fast to shoot (?) based on distance from goal."
            n101 = Wait (ms)(milliseconds to wait=u32 1000) -> ()  [unwired: 1 out]
            n102 = call <vilib>:"WPI_MotorControlSetOutput.vi"("Output"=0.3, "MotorControlDevRef"=w205) -> ()  [unwired: 7 in, 3 out]
          }
          frame #1 {
            # "Window motor spins and feeds frisbees into shooter."
            n103 = call <vilib>:"WPI_MotorControlSetOutput.vi"("Output"=1.0, "MotorControlDevRef"=w208) -> ()  [unwired: 7 in, 3 out]
          }
          frame #2 {
            # "Frisbee Shoots."
            n104 = for {
              N: 3 -> [_]
              # "Frisbee shoots."
              n105 = global read "Robot Global Data.vi" "Shooter Clear"() -> (w213:bool)
              n106 = Not(x=w213) -> (.not. x?=w212:bool)
              n107 = while {
                shift-right: [w215] -> _
                shift-left: FALSE -> [w217]
                tunnel: w212 -> [w215]
                stop <- w214 stop-if-true
                n108 = Not(x=w215) -> (.not. x?=w216:bool)
                n109 = Wait (ms)(milliseconds to wait=u32 10 ("millisecond timer value")) -> ()  [unwired: 1 out]
                n110 = And(x=w216, y=w217) -> (x .and. y?=w214:bool)
              }
            }
          }
          frame #3 {
            # "Window motor and shooter stop after \nall frisbees have been shot."
            n111 = call <vilib>:"WPI_MotorControlSetOutput.vi"("Output"=0.0, "MotorControlDevRef"=w220) -> ()  [unwired: 7 in, 3 out]
            n112 = call <vilib>:"WPI_MotorControlSetOutput.vi"("Output"=0.0, "MotorControlDevRef"=w219) -> ()  [unwired: 7 in, 3 out]
          }
        }
        n113 = global read "Robot Global Data.vi" "Auto Debug"() -> (w198:bool)
        n114 = case shown="True" w198 {
          tunnel: [Auto_States."End" Auto_States."Begin"] -> w202
          frame False {
            # "If Auto Debug is false, then the next state is \"End\""
          }
          frame True {
            # "If Auto Debug is true, then the next state is \"Begin\""
          }
        }
      }
      frame "End" {
        # "If debug false then continues on to next step.\nIf true goes back to debug."
        # "End: If debug false then continues on to next step. If true goes back to debug."
        n115 = global read "Robot Global Data.vi" "Auto Debug"() -> (w224:bool)
        n116 = case shown="True" w224 {
          tunnel: [Auto_States."End" Auto_States."Begin"] -> w226
          frame False {
            # "If Auto Debug is false, then the next state is \"End\""
          }
          frame True {
            # "If Auto Debug is true, then the next state is \"Begin\""
          }
        }
      }
    }
  }
